vi "Scripted Autonomous.vi"   [LabVIEW 2015]
uses:
  Common Code/Shooter Commands.ctl
  Common Code/Shoot Modes Enum.ctl
  Common Code/Change Detect Int.vi
  Robot Global Data.vi
types:
  T1 = typedef "Shoot Modes Enum.ctl" = enum16{"Manual", "Safe", "Auto"}
  T2 = typedef "Shooter Commands.ctl" = enum16{"Idle", "Prime Shooter", "Shoot"}
  T3 = typedef "Dashboard Control Data.ctl" = cluster{"Shooter Presets":T4, "Encoder Control":T6, "Steer PID output":cluster{"output high":dbl, "output low":dbl}, " Steer PID gains":cluster{"proportional gain (Kc)":dbl, "integral time (Ti, min)":dbl, "derivative time (Td, min)":dbl}, "Drivetrain Settings":T7, "Vision Packet":T8, "Dashboard Drivetrain Command":T9, "Info/Command Cluster":T11, "Ball Vision Packet":T12, "Intake Presets":T14, "Intake Encoder Control":T16, "Climb Presets":T17, "Goal Output Range":cluster{"output high":dbl, "output low":dbl}, "Enabled Systems":T18, "Auton Presets":T19, "Pressure M":dbl, "Pressure B":dbl}
  T4 = typedef "Shooter Presets.ctl" = cluster{"Batter Shot":T5, "Deep Middle Shot":T5, "Manual Shot":T5, "Left Ticks Per Rotation":dbl, "Right Ticks Per Rotation":dbl, "Low Bar Shot":T5, "Shooter RPM Tolerance":dbl, "IIR Filter Power":dbl, "Trigger Power":dbl, "Fire from Load Delay":i32, "Max Angle":dbl, "Min Angle":dbl, "Angle PID gains":cluster{"P":dbl, "I":dbl, "D":dbl}, "Angle Output":cluster{"output high":dbl, "output low":dbl}, "Shooter Angle Tolerance":dbl, "Vision Shoot x^2":dbl, "Vision Shoot x":dbl, "Offset Angle":dbl, "High Goal Center Height":dbl, "Feed Forward Max Accel":dbl, "Feed Forward Kv":dbl, "Backwards Trigger":dbl, "Shot Finish Delay (ms)":dbl, "Angle Max Current":dbl, "Angle Current Trip Time":dbl, "Intake Angle":dbl, "Vision Shoot c":dbl, "Reset?":bool, "Servo Release Delay":dbl, "Servo Idle Angle":i32, "Servo Hold Angle":i32, "Angle Pot x":dbl, "Angle Pot c":dbl, "Ignore Angle?":bool, "Manual Output?":bool, "Manual Out":dbl, "Max RPM":dbl, "Safty Frist Angle":dbl, "Intake Danger Height":dbl, "Angle Pot B":i32, "Angle Pot M":dbl, "FF Finish RPM":dbl, "RPM PID Right":cluster{"P":dbl, "I":dbl, "D":dbl, "FF":dbl}, "RPM PID Left":cluster{"P":dbl, "I":dbl, "D":dbl, "FF":dbl}, "Backwards RPM":dbl, "Vision RPM":dbl, "Run Wheels Backward Delay":u32}
  T5 = typedef "Shot Presets.ctl" = cluster{"Left":dbl, "Right":dbl, "Angle":dbl}
  T6 = typedef "Encoder Control.ctl" = cluster{"Right Tick Constant":dbl, "Left Tick Constant":dbl, "Reset?":bool, "Y Dist":cluster{"PID gains":cluster{"proportional gain (Kc)":dbl, "integral time (Ti, min)":dbl, "derivative time (Td, min)":dbl}}, "Y Stop Thresh":dbl, "Y Stop Speed":dbl}
  T7 = typedef "Drivetrain Settings.ctl" = cluster{"Gyro Tolerance":dbl, "Throttle Ramp (ms)":dbl, "Angular rate compensation":bool, "Throttle to Rate Scale":dbl, "Rate compensation gain":dbl, "Kv":dbl, "Ka":dbl, "Feed Forward P":dbl, "Feed Forward D":dbl, "Goal Vision PID gains":cluster{"proportional gain (Kc)":dbl, "integral time (Ti, min)":dbl, "derivative time (Td, min)":dbl}, "Goal Detection Window":dbl, "Creep Rate":dbl}
  T8 = typedef "Goal Vision Packet.ctl" = cluster{"Distance":dbl, "Center X":dbl, "Center Y":dbl, "Found Target?":bool, "Robot Center":dbl, "Angle":dbl}
  T9 = typedef "Dashboard Drivetrain Command.ctl" = cluster{"Drivetrain Vision":T10}
  T10 = typedef "Drivetrain Vision.ctl" = cluster{"Goal Window":dbl, "Ball Window":dbl}
  T11 = typedef "Ball Tracking Command Cluster.ctl" = cluster{"Distance to Ball":dbl, "Desired Angle":dbl, "Command":enum16{"Turn to Ball", "Turn to Angle", "Get Distance"}, "Pixels from Center":dbl}
  T12 = typedef "Ball Vision Packet.ctl" = cluster{"Ball Detected?":bool, "Distance to Ball":dbl, "Desired Angle":dbl, "Pixels from Center":dbl, "Tracking mode":T13}
  T13 = typedef "Tracking Mode.ctl" = enum16{"Turn to Ball", "Turn to Angle"}
  T14 = typedef "Intake Presets.ctl" = cluster{"Intake Speed":dbl, "Outake Speed":dbl, "Low Height":dbl, "Half Height":dbl, "Full Height":dbl, "Angle Speed":dbl, "Angle Tolerance":dbl, "Encoder Scale":dbl, "Load Height":dbl, "Output Range":T15, "Rotation Power Max/Min":dbl, "MaxCurrent":dbl, "Intake Trip Time":dbl, "Idle Height":dbl, "Max Height":dbl, "Reset Encoders?":bool, "PID gains":cluster{"proportional gain (Kc)":dbl, "integral time (Ti, min)":dbl, "derivative time (Td, min)":dbl}, "Intake Stop Delay":u32}
  T15 = typedef "Drivetrain Output Range.ctl" = cluster{"output high":dbl, "output low":dbl}
  T16 = typedef "IntakeEcoderControl.ctl" = cluster{"Arm Tick Constant":dbl, "Reset?":bool, "Y Dist":cluster{"PID gains":cluster{"proportional gain (Kc)":dbl, "integral time (Ti, min)":dbl, "derivative time (Td, min)":dbl}}, "Y Stop Thresh":dbl, "Y Stop Speed":dbl}
  T17 = typedef "Climb Presets.ctl" = cluster{"Pull Power":dbl, "Time to Hold":dbl, "Extend Power":dbl}
  T18 = typedef "Enabled Systems.ctl" = cluster{"Shoot":bool, "Intake":bool, "DT":bool, "Gyro":bool, "100ms":bool, "US":bool}
  T19 = typedef "Autonomous Presets.ctl" = cluster{"Pitch Limit":dbl, "Roll Limit":dbl, "Ultrasonic Limit":dbl, "Start Position":dbl, "Cross Position":dbl}
  T20 = typedef "Auton Command Cluster.ctl" = cluster{"Command ID":i32, "maxTime":dbl, "Y Distance":dbl, "Heading":dbl, "Throttle":dbl, "Async":dbl, "Velocity":dbl, "Acceleration":dbl, "To":dbl, "Condition":dbl, "Shot Type":dbl, "Left RPM":dbl, "Override RPM":i32, "Override Angle":i32, "Right RPM":dbl, "Angle":dbl, "Intake Mode":i32, "Intake Cmd":i32, "Intake O":i32, "Eject O":i32, "Angle O":i32, "Arm O":i32, "Intake Speed":dbl, "Eject Speed":dbl, "Arm Angle":dbl, "Arm Speed":dbl, "Intake?":i32, "Eject?":i32, "Left":dbl, "Right":dbl, "Pivot Speed":dbl, "Y Dist":dbl, "Position":dbl, "Desired Position":i32}
  T21 = typedef "Drivetrain Status Cluster.ctl" = cluster{"Modes":T22, "Y (Throttle)":dbl, "X (Steer)":dbl, "Gyro In Range?":bool, "Distance Drive Finished?":bool, "Stop Eject Lockout":bool, "Dist Drive Status":T23, "Y Target":dbl, "Heading Target":dbl, "Vision Target Aligned?":bool, "Gear":dbl, "1st Gear Time":dbl, "2nd Gear Time":dbl, "1st Gear Shifts":dbl, "2nd Gear Shifts":dbl}
  T22 = typedef "Drivetrain Modes.ctl" = enum16{"Tank", "Climb", "Manual", "Goal Vision Targeting", "PID Distance Drive", "Hybrid", "Gyro Steer"}
  T23 = typedef "Dist Drive Status.ctl" = cluster{"Y In Range":bool, "X In Range":bool, "Gyro In Range":bool, "Y Dist":dbl, "X Dist":dbl, "Gyro":dbl}
  T24 = typedef "Drivetrain Commands.ctl" = cluster{"Y Power":dbl, "Turn Power":dbl, "1st Gear?":bool, "Modes":T22, "Heading Target":dbl, "X Max Speed":dbl, "Y Max Speed":dbl, "X Min Speed":dbl, "Y Min Speed":dbl, "Y Target":dbl, "Max Accel":dbl, "Max Velocity":dbl, "Y Power 2":dbl, "Pivot Speed":dbl}
  T25 = typedef "Shooter Command Cluster.ctl" = cluster{"Command":T2, "Mode":T1, "Shot Type":T26, "Override Trigger Sensor":bool, "Override Angle?":bool, "Hide From Death":bool}
  T26 = typedef "Shot Type.ctl" = enum16{"Batter Shot", "Corner Shot", "Curve Shot", "Vision Shot", "Deep Middle Shot"}
  T27 = typedef "Manual Shoot.ctl" = cluster{"Spin Wheels":bool, "Fire":bool, "Angle":dbl, "Angle Power":dbl, "Use Manual Angle":bool, "Override RPM":bool, "Left RPM":dbl, "Right RPM":dbl, "Secure Ball?":bool}
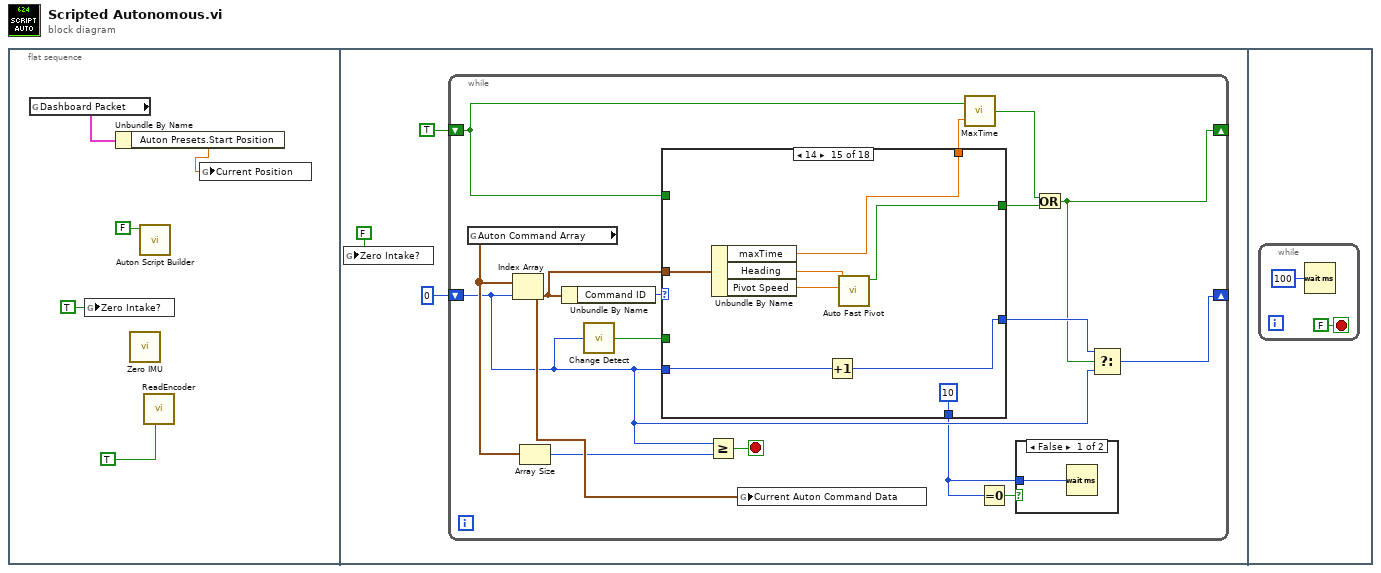
[diagram p0: block diagram]
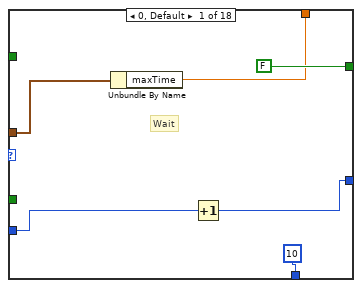
[diagram p3: hidden frame]
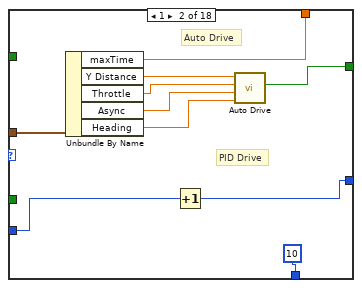
[diagram p4: hidden frame]
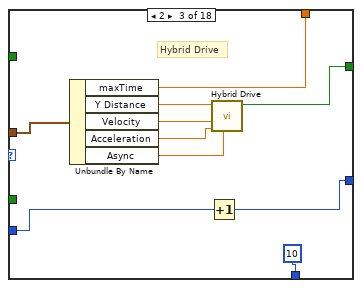
[diagram p5: hidden frame]
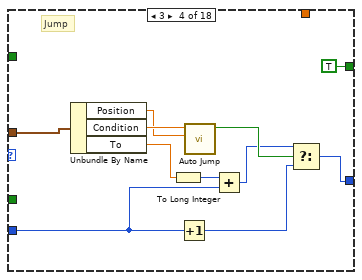
[diagram p6: hidden frame]
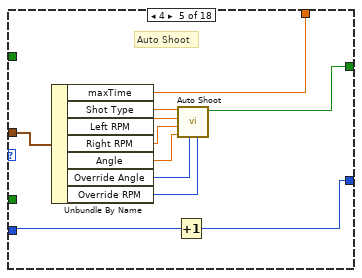
[diagram p7: hidden frame]
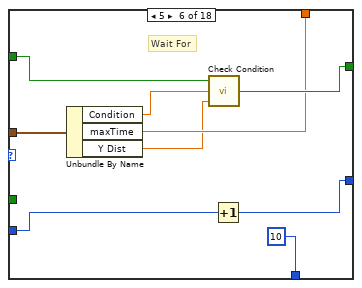
[diagram p8: hidden frame]
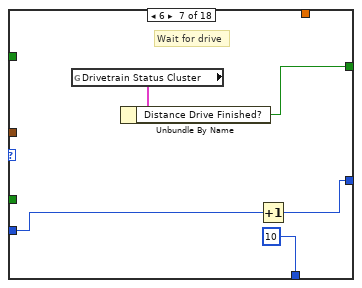
[diagram p9: hidden frame]
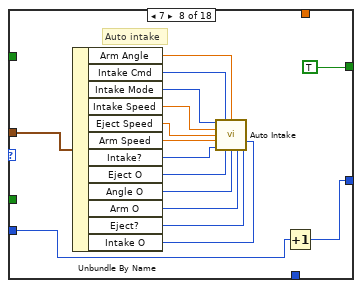
[diagram p10: hidden frame]
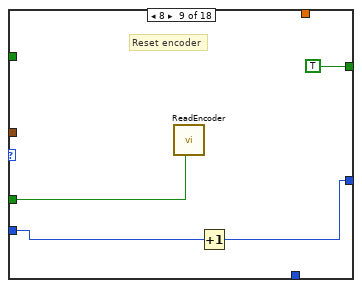
[diagram p11: hidden frame]
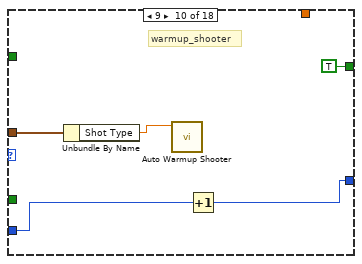
[diagram p12: hidden frame]
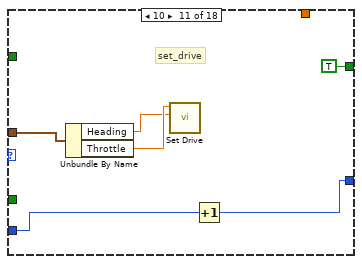
[diagram p13: hidden frame]
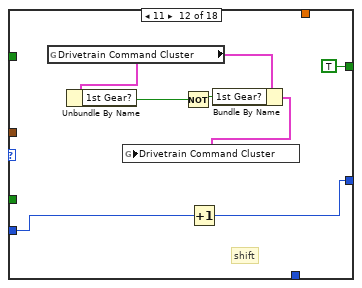
[diagram p14: hidden frame]
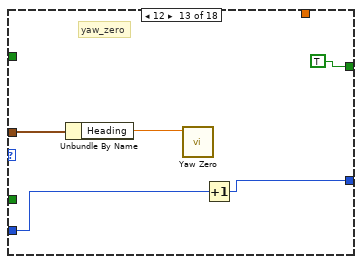
[diagram p15: hidden frame]
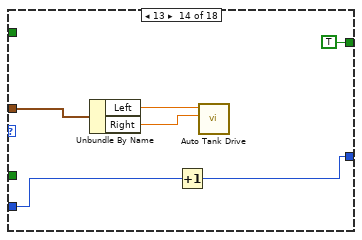
[diagram p16: hidden frame]
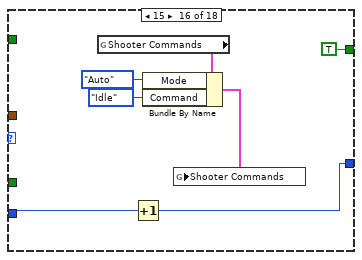
[diagram p17: hidden frame]
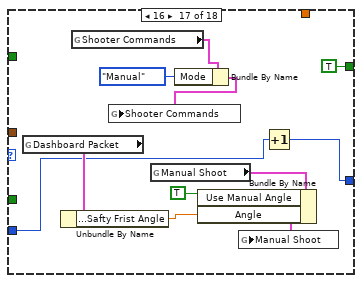
[diagram p18: hidden frame]
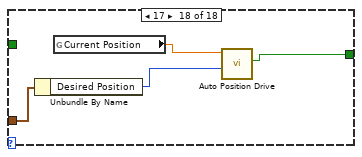
[diagram p19: hidden frame]
diagram:
  n1 = flat-sequence {
    frame #0 {
      n2 = global read "Robot Global Data.vi" "Dashboard Packet"() -> (w2:T3)
      n3 = global write "Robot Global Data.vi" "Zero Intake?"(TRUE ("Zero Intake?")) -> ()
      n4 = Unbundle By Name(w2) -> ("Auton Presets.Start Position"=w1:dbl)
      n5 = call "Zero IMU.vi"() -> ()  [unwired: 12 in]
      n6 = call "Auton Script Builder.vi"("Export?"=FALSE) -> ()  [unwired: 11 in]
      n7 = call "ReadEncoder.vi"("Reset?"=TRUE) -> ()  [unwired: 10 in, 1 out]
      n8 = global write "Robot Global Data.vi" "Current Position"(w1) -> ()
    }
    frame #1 {
      n9 = global write "Robot Global Data.vi" "Zero Intake?"(FALSE ("Zero Intake?")) -> ()
      n10 = while {
        shift-right: [w17] -> _
        shift-left: 0 -> [w18]
        shift-right: [w14] -> _
        shift-left: TRUE -> [w11]
        stop <- w19 stop-if-true
        n11 = global read "Robot Global Data.vi" "Auton Command Array"() -> (w21:T20[])
        n12 = Index Array(array=w21, index=w18) -> (element=w24:T20)
        n13 = Array Size(array=w21) -> (size(s)=w20:i32)
        n14 = Unbundle By Name(w24) -> ("Command ID"=w23:i32)
        n15 = call-poly "Change Detect.vi"("In"=w18) -> ("Changed?"=w22:bool)
        n16 = case shown="14" w23 {
          tunnel: w18 -> [w29 w34 w44 w57 w64 w76 w86 w89 w105 w110 w116 w120 w129 w133 w139 w146 w154 _]
          tunnel: w22 -> [_ _ _ _ _ _ _ _ w107 _ _ _ _ _ _ _ _ _]
          tunnel: w11 -> [_ _ _ _ _ w82 _ _ _ _ _ _ _ _ _ _ _ _]
          tunnel: [w30 w33 w43 w53 w63 w74 w87 w88 w104 w109 w115 w119 w128 w132 w138 w145 w153 _] -> w16
          tunnel: [FALSE w35 w47 TRUE ("Distance Drive Finished?") w65 w81 w85 TRUE TRUE ("Distance Drive Finished?") TRUE ("Distance Drive Finished?") TRUE ("Distance Drive Finished?") TRUE ("Distance Drive Finished?") TRUE TRUE ("Distance Drive Finished?") w141 TRUE ("Done?") TRUE ("Done?") w163] -> w15
          tunnel: [w27 w40 w45 _ w66 w79 _ _ _ _ _ _ _ _ w140 _ _ _] -> w12
          tunnel: w24 -> [w28 w41 w51 w61 w73 w77 _ w102 _ w112 w118 _ w127 w136 w144 _ _ w166]
          tunnel: [10 10 10 _ _ 10 10 _ _ _ _ _ _ _ 10 _ _ _] -> w10
          frame 0, Default {
            # "Wait"
            n17 = Unbundle By Name(w28) -> ("maxTime"=w27:dbl)
            n18 = Increment(x=w29) -> (x+1=w30:i32)
          }
          frame 1 {
            # "Auto Drive"
            # "PID Drive"
            n19 = Unbundle By Name(w41) -> ("maxTime"=w40:dbl, "Y Distance"=w39:dbl, "Throttle"=w38:dbl, "Async"=w37:dbl, "Heading"=w36:dbl)
            n20 = Increment(x=w34) -> (x+1=w33:i32)
            n21 = call "Auto Drive.vi"("heading"=w36, "async"=w37, "speed"=w38, "y"=w39) -> ("isFinished?"=w35:bool)  [unwired: 7 in]
          }
          frame 2 {
            # "Hybrid Drive"
            n22 = Unbundle By Name(w51) -> ("maxTime"=w45:dbl, "Y Distance"=w50:dbl, "Velocity"=w49:dbl, "Acceleration"=w48:dbl, "Async"=w46:dbl)
            n23 = Increment(x=w44) -> (x+1=w43:i32)
            n24 = call "Hybrid Drive.vi"("Async?"=w46, "Max Accel"=w48, "Max Velocity"=w49, "Distance"=w50) -> ("Finished?"=w47:bool)  [unwired: 7 in]
          }
          frame 3 {
            # "Jump"
            n25 = Unbundle By Name(w61) -> ("Position"=w52:dbl, "Condition"=w60:dbl, "To"=w55:dbl)
            n26 = To Long Integer(number=w55) -> (32bit integer=w56:i32)
            n27 = Increment(x=w57) -> (x+1=w58:i32)
            n28 = call "Auto Jump.vi"("Position"=w52, "Condition"=w60) -> ("Jump?"=w59:bool)  [unwired: 9 in]
            n29 = Add(x=w56, y=w57) -> (x+y=w54:i32)
            n30 = Select(t=w54, s=w59, f=w58) -> (s? t:f=w53:i32)
          }
          frame 4 {
            # "Auto Shoot"
            n31 = Unbundle By Name(w73) -> ("maxTime"=w66:dbl, "Shot Type"=w72:dbl, "Left RPM"=w71:dbl, "Right RPM"=w70:dbl, "Angle"=w69:dbl, "Override Angle"=w68:i32, "Override RPM"=w67:i32)
            n32 = Increment(x=w64) -> (x+1=w63:i32)
            n33 = call "Auto Shoot.vi"("RPM Override?"=w67, "Angle Override?"=w68, "Angle"=w69, "Right RPM"=w70, "Left RPM"=w71, "Shot Type"=w72) -> ("Finished?"=w65:bool)  [unwired: 5 in]
          }
          frame 5 {
            # "Wait For"
            n34 = Unbundle By Name(w77) -> ("Condition"=w80:dbl, "maxTime"=w79:dbl, "Y Dist"=w78:dbl)
            n35 = call "Check Condition.vi"("Distance"=w78, "Condition"=w80, "Reset"=w82) -> ("Done"=w81:bool)
            n36 = Increment(x=w76) -> (x+1=w74:i32)
          }
          frame 6 {
            # "Wait for drive"
            n37 = global read "Robot Global Data.vi" "Drivetrain Status Cluster"() -> (w84:T21)
            n38 = Unbundle By Name(w84) -> ("Distance Drive Finished?"=w85:bool)
            n39 = Increment(x=w86) -> (x+1=w87:i32)
          }
          frame 7 {
            # "Auto intake"
            n40 = Unbundle By Name(w102) -> ("Arm Angle"=w101:dbl, "Intake Cmd"=w100:i32, "Intake Mode"=w99:i32, "Intake Speed"=w98:dbl, "Eject Speed"=w97:dbl, "Arm Speed"=w96:dbl, "Intake?"=w95:i32, "Eject O"=w94:i32, "Angle O"=w93:i32, "Arm O"=w92:i32, "Eject?"=w91:i32, "Intake O"=w90:i32)
            n41 = call "Auto Intake.vi"("Intake Mode ID"=w99, "Intake Command ID"=w100, "Arm Angle"=w101, "Intake Override Speed"=w98, "Eject Override Speed"=w97, "Arm Speed"=w96, "Override Intake?"=w90, "Intake?"=w95, "Override Eject?"=w94, "Override Angle?"=w93, "Override Arm?"=w92, "Eject?"=w91) -> ()  [unwired: 4 in]
            n42 = Increment(x=w89) -> (x+1=w88:i32)
          }
          frame 8 {
            # "Reset encoder"
            n43 = call "ReadEncoder.vi"("Reset?"=w107) -> ()  [unwired: 10 in, 1 out]
            n44 = Increment(x=w105) -> (x+1=w104:i32)
          }
          frame 9 {
            # "warmup_shooter"
            n45 = Unbundle By Name(w112) -> ("Shot Type"=w111:dbl)
            n46 = call "Auto Warmup Shooter.vi"("Shot Type"=w111) -> ()  [unwired: 11 in]
            n47 = Increment(x=w110) -> (x+1=w109:i32)
          }
          frame 10 {
            # "set_drive"
            n48 = Unbundle By Name(w118) -> ("Heading"=w113:dbl, "Throttle"=w114:dbl)
            n49 = call "Set Drive.vi"("Heading Target"=w113, "Y Power"=w114) -> ()  [unwired: 10 in]
            n50 = Increment(x=w116) -> (x+1=w115:i32)
          }
          frame 11 {
            # "shift"
            n51 = global read "Robot Global Data.vi" "Drivetrain Command Cluster"() -> (w125:T24)
            n52 = Unbundle By Name(w125) -> ("1st Gear?"=w124:bool)
            n53 = Not(x=w124) -> (.not. x?=w123:bool)
            n54 = Increment(x=w120) -> (x+1=w119:i32)
            n55 = Bundle By Name(cluster=w125, "1st Gear?"=w123) -> (w122:T24)
            n56 = global write "Robot Global Data.vi" "Drivetrain Command Cluster"(w122) -> ()
          }
          frame 12 {
            # "yaw_zero"
            n57 = Unbundle By Name(w127) -> ("Heading"=w126:dbl)
            n58 = call "Yaw Zero.vi"("Angle"=w126) -> ()  [unwired: 11 in]
            n59 = Increment(x=w129) -> (x+1=w128:i32)
          }
          frame 13 {
            n60 = Unbundle By Name(w136) -> ("Left"=w135:dbl, "Right"=w134:dbl)
            n61 = Increment(x=w133) -> (x+1=w132:i32)
            n62 = call "Auto Tank Drive.vi"("Right"=w134, "Left"=w135) -> ()  [unwired: 10 in]
          }
          frame 14 {
            n63 = Unbundle By Name(w144) -> ("maxTime"=w140:dbl, "Heading"=w142:dbl, "Pivot Speed"=w143:dbl)
            n64 = Increment(x=w139) -> (x+1=w138:i32)
            n65 = call "Auto Fast Pivot.vi"("Pivot Speed"=w143, "Heading"=w142) -> ("Done?"=w141:bool)  [unwired: 9 in]
          }
          frame 15 {
            n66 = global read "Robot Global Data.vi" "Shooter Commands"() -> (w151:T25)
            n67 = Increment(x=w146) -> (x+1=w145:i32)
            n68 = Bundle By Name(cluster=w151, "Mode"=Shoot_Modes_Enum."Auto", "Command"=Shooter_Commands."Idle") -> (w148:T25)
            n69 = global write "Robot Global Data.vi" "Shooter Commands"(w148) -> ()
          }
          frame 16 {
            n70 = global read "Robot Global Data.vi" "Dashboard Packet"() -> (w156:T3)
            n71 = Unbundle By Name(w156) -> ("Shooter Presets.Safty Frist Angle"=w155:dbl)
            n72 = global read "Robot Global Data.vi" "Shooter Commands"() -> (w162:T25)
            n73 = global read "Robot Global Data.vi" "Manual Shoot"() -> (w159:T27)
            n74 = Bundle By Name(cluster=w162, "Mode"=Shoot_Modes_Enum."Manual") -> (w160:T25)
            n75 = global write "Robot Global Data.vi" "Shooter Commands"(w160) -> ()
            n76 = Bundle By Name(cluster=w159, "Use Manual Angle"=TRUE, "Angle"=w155) -> (w158:T27)
            n77 = global write "Robot Global Data.vi" "Manual Shoot"(w158) -> ()
            n78 = Increment(x=w154) -> (x+1=w153:i32)
          }
          frame 17 {
            n79 = Unbundle By Name(w166) -> ("Desired Position"=w164:i32)
            n80 = global read "Robot Global Data.vi" "Current Position"() -> (w165:dbl)
            n81 = call "Auto Position Drive.vi"("Desired Position"=w164, "Current Position"=w165) -> ("Finished?"=w163:bool)  [unwired: 9 in]
          }
        }
        n82 = Greater Or Equal?(x=w18, y=w20) -> (x >= y?=w19:bool)
        n83 = global write "Robot Global Data.vi" "Current Auton Command Data"(w24) -> ()
        n84 = call "MaxTime.vi"("MaxTime"=w12, "Reset?"=w11) -> ("Finished?"=w13:bool)
        n85 = Equal To 0?(x=w10) -> (x = 0?=w9:bool)
        n86 = case shown="False" w9 {
          tunnel: w10 -> [w25 _]
          frame False {
            n87 = Wait (ms)(milliseconds to wait=w25) -> ()  [unwired: 1 out]
          }
          frame True {
          }
        }
        n88 = Or(x=w13, y=w15) -> (x .or. y?=w14:bool)
        n89 = Select(t=w16, s=w14, f=w18) -> (s? t:f=w17:i32)
      }
    }
    frame #2 {
      n90 = while {
        stop <- FALSE stop-if-true
        n91 = Wait (ms)(milliseconds to wait=u32 100) -> ()  [unwired: 1 out]
      }
    }
  }
